vi "Test Biosemi TCP Thread.vi"() -> (15 "error out":errorcluster)   [LabVIEW 2016]
panel:
  out "graph":dbl[][](graph)
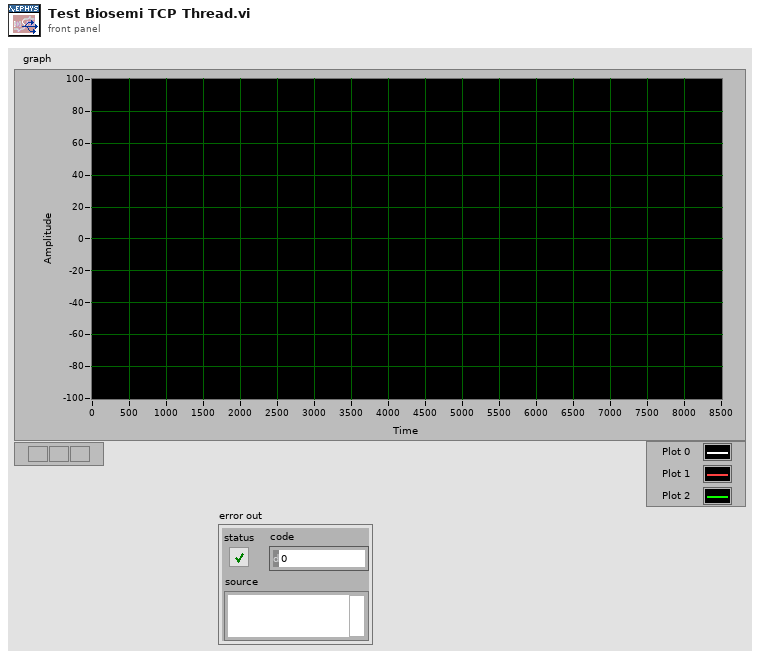
[diagram p1: front panel]
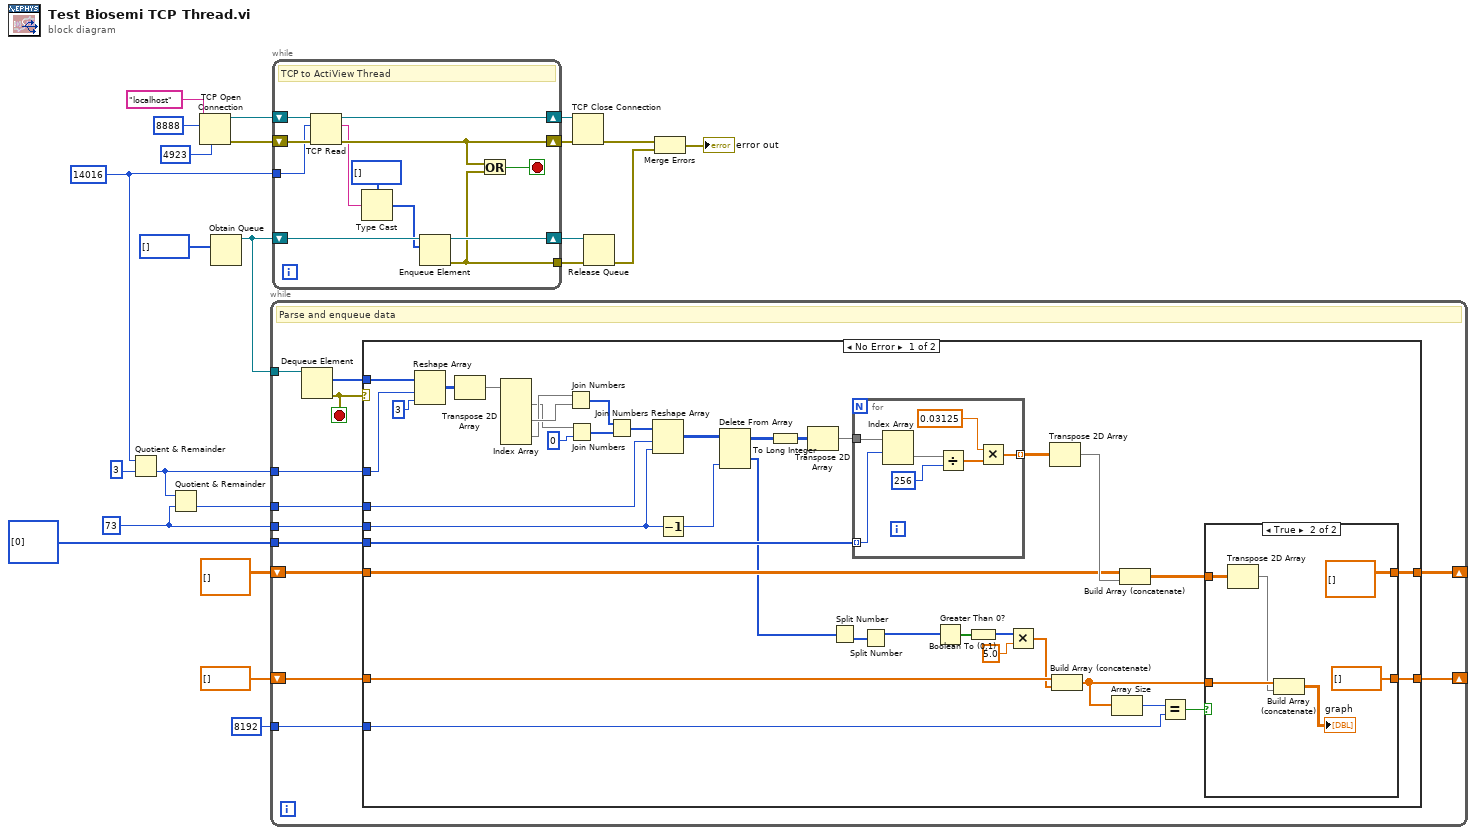
[diagram p0: block diagram]
diagram:
  w3 = 73
  w4 = 14016 ("value")
  n1 = Quotient & Remainder(x=w4, y=3) -> (floor(x/y)=w8:i32)  [unwired: 1 out]
  n2 = Quotient & Remainder(x=w8, y=w3) -> (floor(x/y)=w7:i32)  [unwired: 1 out]
  n3 = TCP Open Connection(address="localhost", remote port or service name=u16 8888, local port=u16 4923 ("local port (0)")) -> (connection ID=w19:refnum<k5>, error out=w18:errorcluster)  [unwired: 2 in]
  n4 = Obtain Queue(element data type=u8[] []) -> (queue out=w11:refnum<queue>)  [unwired: 4 in, 2 out]
  n5 = while {
    tunnel: w11 -> [w35]
    shift-right: [w31] -> _
    shift-left: dbl[][] [] ("output array") -> [w32]
    tunnel: w8 -> [w30]
    tunnel: w3 -> [w29]
    tunnel: w7 -> [w28]
    tunnel: i32[] [0] ("keep") -> [w27]
    shift-right: [w25] -> _
    shift-left: dbl[] [] ("output array") -> [w26]
    tunnel: 8192 ("Sample rate") -> [w24]
    stop <- w34 stop-if-true
    # "Parse and enqueue data"
    n6 = Dequeue Element(queue=w35) -> (element=w33:u8[], error out=w34:errorcluster)  [unwired: 2 in, 2 out]
    n7 = case shown="No Error" w34 {
      tunnel: w33 -> [w63 _]
      tunnel: w32 -> [w53 w90]
      tunnel: [w73 w90] -> w31
      tunnel: w30 -> [w62 _]
      tunnel: w29 -> [w60 _]
      tunnel: w28 -> [w52 _]
      tunnel: w27 -> [w56 _]
      tunnel: w26 -> [w48 w89]
      tunnel: [w41 w89] -> w25
      tunnel: w24 -> [w45 _]
      frame No Error {
        n8 = Reshape Array(w63, w62, 3) -> (w69:u8[][])
        n9 = Transpose 2D Array(2D array=w69) -> (transposed array=w65:u8[][])
        n10 = Index Array(array=w65) -> (element #1=w40:u8[], element #2=w71:u8[], element #3=w70:u8[])  [unwired: 6 in]
        n11 = Join Numbers(hi=w70, lo=w71) -> ((hi.lo)=w66:u16[])
        n12 = Join Numbers(hi=w40, lo=u8 0) -> ((hi.lo)=w67:u16[])
        n13 = Join Numbers(hi=w66, lo=w67) -> ((hi.lo)=w64:u32[])
        n14 = Reshape Array(w64, w52, w60) -> (w61:u32[][])
        n15 = Decrement(x=w60) -> (x-1=w59:i32)
        n16 = Delete From Array(array=w61, index (col)=w59) -> (deleted portion=w39:u32[], array with subset deleted=w58:u32[][])  [unwired: 2 in]
        n17 = To Long Integer(number=w58) -> (32bit integer=w36:i32[][])
        n18 = Transpose 2D Array(2D array=w36) -> (transposed array=w57:i32[][])
        n19 = Split Number(x=w39) -> (lo(x)=w38:u16[])  [unwired: 1 out]
        n20 = for {
          tunnel: w57 -> [w80]
          tunnel: w56 -> [w79] mode=indexing
          tunnel: [w74] -> w55 mode=indexing
          n21 = Index Array(array=w80, index (row)=w79) -> (element=w78:i32[])  [unwired: 1 in]
          n22 = Divide(x=w78, y=256) -> (x/y=w75:dbl[])
          n23 = Multiply(x=0.03125, y=w75) -> (x*y=w74:dbl[])
        }
        n24 = Split Number(x=w38) -> (hi(x)=w37:u8[])  [unwired: 1 out]
        n25 = Greater Than 0?(x=w37) -> (x > 0?=w51:bool[])
        n26 = Boolean To (0,1)(Boolean=w51) -> (0, 1=w50:i16[])
        n27 = Multiply(x=w50, y=5.0) -> (x*y=w47:dbl[])
        n28 = Transpose 2D Array(2D array=w55) -> (transposed array=w54:dbl[][])
        n29 = Build Array (concatenate)(w48, w47) -> (w43:dbl[])
        n30 = Array Size(array=w43) -> (size(s)=w46:i32)
        n31 = Build Array (concatenate)(w53, w54) -> (w42:dbl[][])
        n32 = Equal?(x=w46, y=w45) -> (x = y?=w44:bool)
        n33 = case shown="True" w44 {
          tunnel: [w82 dbl[][] [] ("output array")] -> w73
          tunnel: w43 -> [w81 w85]
          tunnel: w42 -> [w82 w86]
          tunnel: [w81 dbl[] []] -> w41
          frame False {
          }
          frame True {
            n34 = Transpose 2D Array(2D array=w86) -> (transposed array=w84:dbl[][])
            n35 = Build Array (concatenate)(w85, w84) -> (→"graph":dbl[][])
          }
        }
      }
      frame Error {
      }
    }
  }
  n36 = while {
    shift-right: [w98] -> w20
    shift-left: w18 -> [w102]
    shift-right: [w101] -> w21
    shift-left: w19 -> [w100]
    tunnel: w4 -> [w99]
    shift-right: [w94] -> w14
    shift-left: w11 -> [w95]
    tunnel: [w93] -> w13
    stop <- w91 stop-if-true
    # "TCP to ActiView Thread"
    n37 = TCP Read(connection ID=w100, bytes to read=w99, error in (no error)=w102) -> (connection ID out=w101:refnum<k5>, data out=w96:string, error out=w98:errorcluster)  [unwired: 2 in]
    n38 = Type Cast(type=u8[] [], x=w96) -> (*(type *) &x=w92:u8[])
    n39 = Enqueue Element(queue=w95, element=w92) -> (queue out=w94:refnum<queue>, error out=w93:errorcluster)  [unwired: 2 in, 1 out]
    n40 = Or(x=w98, y=w93) -> (x .or. y?=w91:bool)
  }
  n41 = TCP Close Connection(connection ID=w21, error in (no error)=w20) -> (error out=w17:errorcluster)  [unwired: 1 in, 1 out]
  n42 = Release Queue(queue=w14, error in (no error)=w13) -> (error out=w12:errorcluster)  [unwired: 1 in, 2 out]
  n43 = Merge Errors(w17, w12) -> (→"error out":errorcluster)
